vi "Actor Core.vi"(8 "error in":errorcluster, 11 "RandomDataChart in":refnum<class "RandomDataChart.lvclass">) -> (0 "error out":errorcluster, 3 "Actor out":refnum<class "Actor.lvclass">)   [LabVIEW 2015, in "TestViewables.lvlib" / "RandomDataChart.lvclass"]
doc: "(<B>Filename</B>: Actor Framework.lvlib:Actor.lvclass:Actor Core.vi)\n\nReceives messages to the actor, reacts to them, and initiates any error handling that may shut the actor down.\n\nDescendant classes may override this VI to append parallel tasks for the actor to complete while it handles messages. Overrides use the Call Parent Method node.\n\n<License>\nCopyright © 2017 Composed Systems, LLC | All rights reserved\nwww.composed.io\n\nAuthor: Ethan Stern <ethan.stern@composed.io>\n\nThis software is provided \"AS IS\" WITHOUT WARRANTIES, either express or implied, AND IS FOR EDUCATIONAL PURPOSES ONLY.\n</License>"
uses:
  RandomDataChart.lvclass
  <vilib>/ActorFramework/Actor/Actor.lvclass
  Framework/IViewable/IViewable/IViewable.lvclass
  Framework/IObserver/IObserver/IObserver.lvclass
panel:
  out "Random Number":dbl(graph)
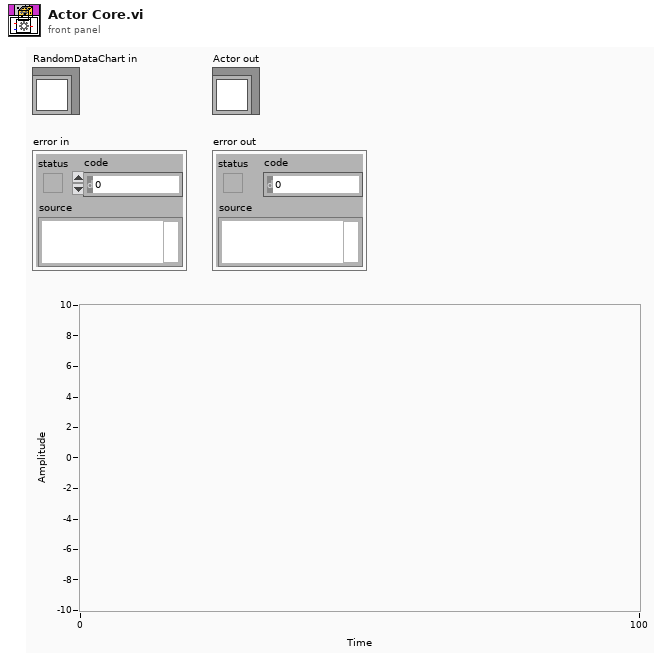
[diagram p1: front panel]
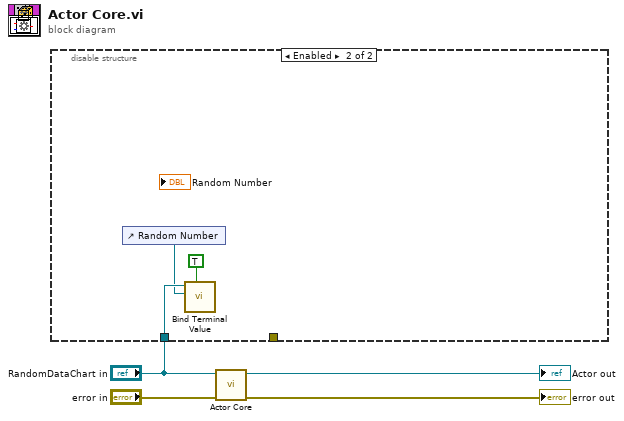
[diagram p0: block diagram]
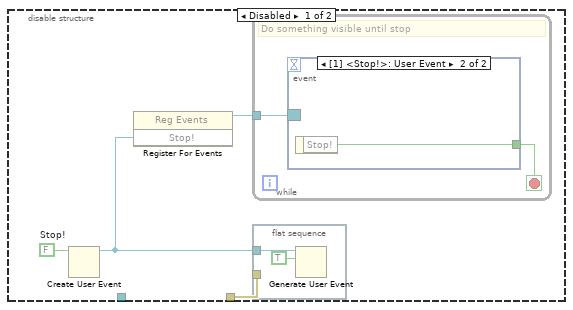
[diagram p2: hidden frame]
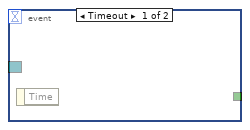
[diagram p3: hidden frame]
diagram:
  n1 = disable-structure shown="Enabled" {
    disable-tunnel: _ -> [w7 _]
    disable-tunnel: "RandomDataChart in" -> [_ w16]
    frame Disabled {
      w8 = FALSE  # Stop!
      n2 = Create User Event(user event datatype=w8) -> (user event=w5:refnum<user-event>)  [unwired: 1 in, 1 out]
      n3 = register-events(w5) -> (reference out=w6:refnum<event-registration>)  [unwired: 2 in, 1 out]
      n4 = while {
        tunnel: w6 -> [w12]
        stop <- w11 stop-if-true
        # "Do something visible until stop"
        n5 = event shown="[1] <Stop!>: User Event" {
          selector: w12 -> [_ _]
          dyn-events: _ -> [_ _]
          timeout: _ -> [_ _]
          tunnel: [_ w13] -> w11
          event Timeout {
            n6 = event-data() -> ()  [unwired: 1 in, 1 out]
          }
          event User Event {
            n7 = event-data() -> ("Stop!"=w13:bool)  [unwired: 1 in]
          }
        }
      }
      n8 = flat-sequence {
        tunnel: w5 -> [w10]
        tunnel: w7 -> [_]
        frame #0 {
          n9 = Generate User Event(user event=w10, event data cluster=TRUE ("event data")) -> ()  [unwired: 2 in, 2 out]
        }
      }
    }
    frame Enabled {
      n10 = control-ref of="Random Number"() -> (w15:refnum<vi>)
      n11 = call "Bind Terminal Value.vi"("Bind by Label (F=Bind by Caption)"=TRUE ("Use Label Text (F=Use Caption)"), "Ctl Refnum"=w15, "IObserver in"=w16) -> ()  [unwired: 7 in, 2 out]
    }
  }
  n12 = call-parent "Actor Core.vi"("error in"="error in", "IViewable In"="RandomDataChart in") -> ("error out"=→"error out":errorcluster, "Actor out"=→"Actor out":refnum<class "Actor.lvclass">)  [unwired: 8 in]
